vi "TX example.vi"() -> ()   [LabVIEW 2010]
uses:
  <vilib>/Analysis/2dsp.llb/Complex FFT.vi
  <vilib>/Analysis/NI_AALPro.lvlib
panel:
  out "S(t)":dbl[](graph)
  out "S(w)":dbl[](graph)
  in  "CarrierFreqHz":dbl(slide)=90658509.45494995 scale=86000000.0..110000000.0 scale format="%#_6p"
  in  "VGAGainDb":dbl=20.0 min=0.0 max=62.0 step=2.0
  in  "stop":bool
  in  "SampleFreqHz":dbl=4500000.0 format="%#_6p"
  in  "FilterBandwidthHz":dbl=3000000.0 format="%#_6p"
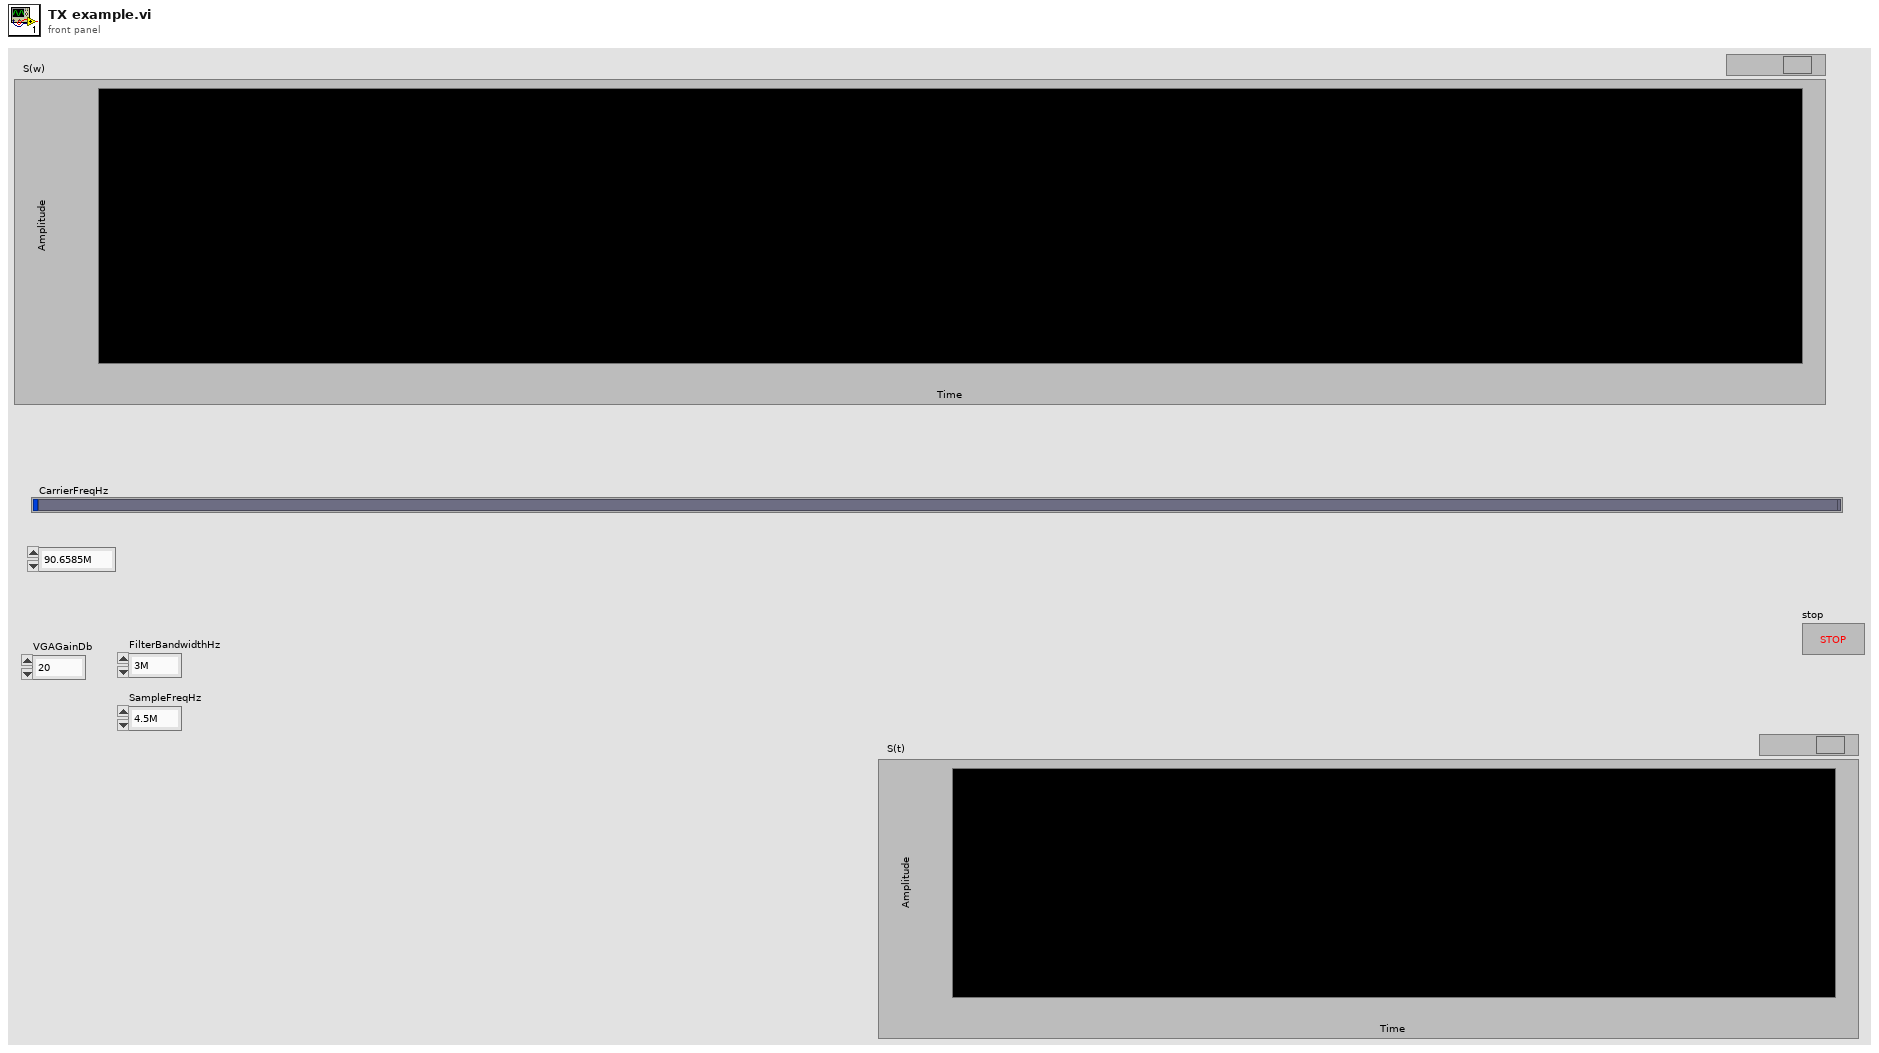
[diagram p1: front panel]
types:
  T1 = typedef "HackRF_Ref.ctl" = cluster{".net":refnum<k24>, "HackrfDeviceList":refnum<k24>[], "OpenDevice":refnum<k24>, "StartRX":refnum<k24>, "CarrierFreqHz":dbl, "SampleFreqHz":dbl, "FilterBandwidthHz":dbl, "AMPEnable":bool, "LNAGainDb":dbl, "VGAGainDb":dbl, "StartTx":refnum<k24>}
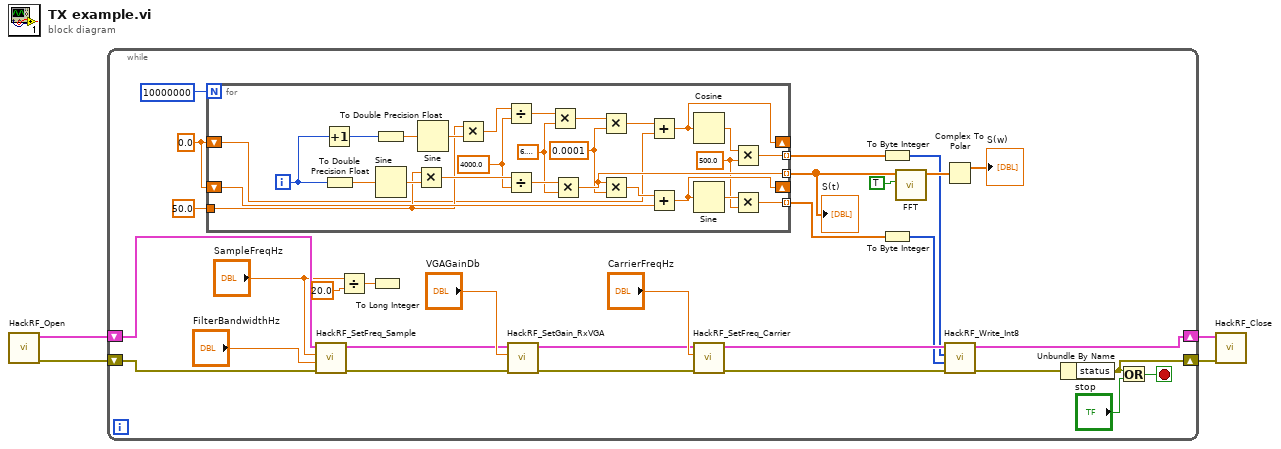
[diagram p0: block diagram]
diagram:
  n1 = call "HackRF_Open.vi"() -> ("error out"=w3:errorcluster, "Cluster"=w4:T1)  [unwired: 10 in]
  n2 = while {
    shift-right: [w20] -> w2
    shift-left: w4 -> [w34]
    shift-right: [w19] -> w1
    shift-left: w3 -> [w33]
    stop <- w24 stop-if-true
    w16 = 0.0
    n3 = for {
      N: 10000000 -> [_]
      tunnel: 50.0 -> [w47]
      shift-right: [w53] -> _
      shift-left: w16 -> [w57]
      tunnel: [w56] -> w10 mode=indexing
      tunnel: [w52] -> w6 mode=indexing
      shift-right: [w40] -> _
      shift-left: w16 -> [w42]
      tunnel: [w39] -> w7 mode=indexing
      i -> [w51]
      w38 = 500.0 ("y")
      w37 = 0.0001 ("y")
      w36 = 6.283185307179586
      w35 = 4000.0 ("y")
      n4 = Increment(x=w51) -> (x+1=w49:i32)
      n5 = To Double Precision Float(number=w51) -> (double precision float=w61:dbl)
      n6 = To Double Precision Float(number=w49) -> (double precision float=w50:dbl)
      n7 = Sine(x=w61) -> (sin(x)=w60:dbl)
      n8 = Multiply(x=w47, y=w60) -> (x*y=w59:dbl)
      n9 = Sine(x=w50) -> (sin(x)=w48:dbl)
      n10 = Multiply(x=w47, y=w48) -> (x*y=w46:dbl)
      n11 = Divide(x=w46, y=w35) -> (x/y=w45:dbl)
      n12 = Divide(x=w59, y=w35) -> (x/y=w58:dbl)
      n13 = Multiply(x=w45, y=w36) -> (x*y=w44:dbl)
      n14 = Multiply(x=w58, y=w36) -> (x*y=w56:dbl)
      n15 = Multiply(x=w44, y=w37) -> (x*y=w43:dbl)
      n16 = Multiply(x=w56, y=w37) -> (x*y=w55:dbl)
      n17 = Add(x=w43, y=w42) -> (x+y=w40:dbl)
      n18 = Add(x=w55, y=w57) -> (x+y=w53:dbl)
      n19 = Cosine(x=w40) -> (cos(x)=w41:dbl)
      n20 = Sine(x=w53) -> (sin(x)=w54:dbl)
      n21 = Multiply(x=w41, y=w38) -> (x*y=w39:dbl)
      n22 = Multiply(x=w54, y=w38) -> (x*y=w52:dbl)
    }
    "S(t)" <- w10
    n23 = call "HackRF_SetFreq_Sample.vi"("error in (no error)"=w33, "FilterBandwidthHz"="FilterBandwidthHz", "SampleFreqHz"="SampleFreqHz", "HackRF in"=w34) -> ("error out"=w13:errorcluster, "HackRF out"=w14:T1)  [unwired: 6 in]
    n24 = Divide(x="SampleFreqHz", y=20.0) -> (x/y=w30:dbl)
    n25 = To Long Integer(number=w30) -> ()  [unwired: 1 out]
    n26 = call "HackRF_SetGain_RxVGA.vi"("error in (no error)"=w13, "VGAGainDb"="VGAGainDb", "HackRF in"=w14) -> ("error out"=w11:errorcluster, "HackRF out"=w12:T1)  [unwired: 7 in]
    n27 = call "HackRF_SetFreq_Carrier.vi"("error in (no error)"=w11, "CarrierFreqHz"="CarrierFreqHz", "HackRF_In"=w12) -> ("error out"=w21:errorcluster, "HackRF_Out"=w22:T1)  [unwired: 7 in]
    n28 = To Byte Integer(number=w7) -> (8bit integer=w9:i8[])
    n29 = To Byte Integer(number=w6) -> (8bit integer=w8:i8[])
    n30 = call-poly <vilib>:"FFT.vi"("shift?"=TRUE, "X"=w10) -> ("FFT {X}"=w26:cdb[])  [unwired: 8 in, 1 out]
    n31 = Complex To Polar(r * e^(i*theta)=w26) -> (r=→"S(w)":dbl[])  [unwired: 1 out]
    n32 = call "HackRF_Write_Int8.vi"("error in (no error)"=w21, "Q data"=w8, "I data"=w9, "HackRF"=w22) -> ("error out"=w19:errorcluster, "HackRF"=w20:T1)  [unwired: 6 in]
    n33 = Unbundle By Name(w19) -> ("status"=w5:bool)
    n34 = Or(x=w5, y="stop") -> (x .or. y?=w24:bool)
  }
  n35 = call "HackRF_Close.vi"("error in (no error)"=w1, "Cluster in"=w2) -> ()  [unwired: 8 in, 2 out]
